vi "Rotation_CreateAngleRotations.vi"(11 "Angle_Rotations":dbl) -> (3 "ROTATION":T1 {"SIN" format="%13.4f"; "COS" format="%13.4f"; "VALUE" format="%13.4f"})   [LabVIEW 2019, in "Trajectory_Library.lvlib"]
doc: "Constructs a Rotation2d with the given angle value in rotations.\nParmeters:\n - value - The value of the angle in rotations.\n\nReturns\n - rotation data structure"
uses:
  ROTATION2D.ctl
  Trajectory_Library.lvlib
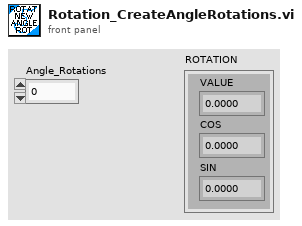
[diagram p1: front panel]
types:
  T1 = typedef "Trajectory_Library.lvlib/ROTATION2D.ctl" = cluster{"VALUE":dbl, "COS":dbl, "SIN":dbl}
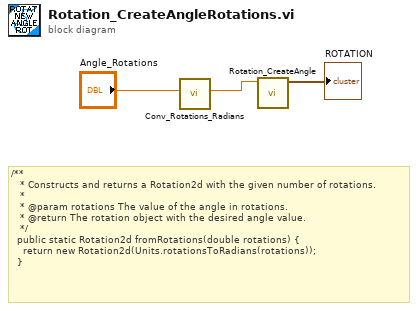
[diagram p0: block diagram]
diagram:
  # "/**\n   * Constructs and returns a Rotation2d with the given number of rotations.\n   *\n   * @param rotations The value of the angle in rotations.\n   * @return The rotation object with the desired angle value.\n   */\n  public static Rotation2d fromRotations(double rotations) {\n    return new Rotation2d(Units.rotationsToRadians(rotations));\n  }"
  n1 = call "Conv_Rotations_Radians.vi"("Rotations"="Angle_Rotations") -> ("Radians"=w1:dbl)  [unwired: 10 in]
  n2 = call "Rotation_CreateAngle.vi"("Angle"=w1) -> ("ROTATION"=→"ROTATION":T1)  [unwired: 10 in]
